vi "StringFunctions_ReplaceAllBlindSigns.vi"(0 "String":string, 3 "RemoveSpaceAswell":bool, 5 "ErrorIn":errorcluster) -> (14 "ModifiedString":string, 19 "ErrorOut":errorcluster)   [LabVIEW 2016]
doc: "Entfernt alle EOL, CR usw. Zeichen. Space optional, default = F\n\n22.04.14 / sige"
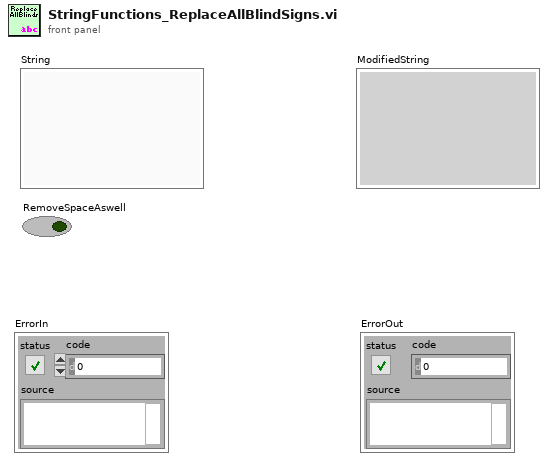
[diagram p1: front panel]
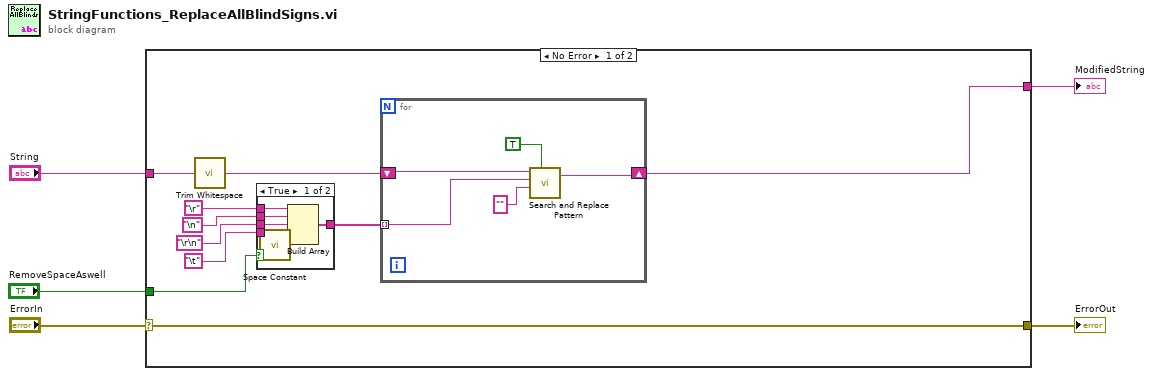
[diagram p0: block diagram]
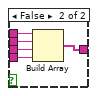
[diagram p2: hidden frame]
diagram:
  n1 = case shown="No Error" "ErrorIn" {
    selector: "ErrorIn" -> [w7 w33]
    tunnel: [w7 w33] -> w4
    tunnel: "String" -> [w15 w32]
    tunnel: [w6 w32] -> w2
    tunnel: "RemoveSpaceAswell" -> [w8 _]
    frame No Error {
      n2 = call <vilib>:"Trim Whitespace.vi"("string"=w15) -> ("trimmed string"=w14:string)  [unwired: 1 in]
      n3 = case shown="True" w8 {
        tunnel: "\r" -> [w21 w26]
        tunnel: "\n" -> [w20 w25]
        tunnel: "\r\n" -> [w19 w24]
        tunnel: "\t" -> [w18 w23]
        tunnel: [w16 w22] -> w9
        frame True {
          n4 = call <vilib>:"Space Constant.vi"() -> ("String"=w17:string)
          n5 = Build Array(w21, w20, w19, w18, w17) -> (w16:string[])
        }
        frame False {
          n6 = Build Array(w26, w25, w24, w23) -> (w22:string[])
        }
      }
      n7 = for {
        shift-right: [w29] -> w6
        shift-left: w14 -> [w31]
        tunnel: w9 -> [w27] mode=indexing
        n8 = call <vilib>:"Search and Replace Pattern.vi"("string"=w31, "regular expression (\"\")"=w27, "replace string (\"\")"="" ("replace string (\"\")"), "replace all? (F)"=TRUE) -> ("result string"=w29:string)  [unwired: 1 in, 1 out]
      }
    }
    frame Error {
    }
  }
  "ErrorOut" <- w4
  "ModifiedString" <- w2
